vi "CLD3 FGV Timer Exercise.vi"(8 "Fehler (Eingang)":T1, 10 "Zielzeit (s)":dbl, 11 "Timer-Modus":T2) -> (0 "Fehler (Ausgang)":T1, 3 "Verstrichene Zeit (s,ms)":dbl)   [LabVIEW 2009]
doc: "CLD-Übung 3"
uses:
  CLD3 FGV Mode.ctl
panel:
  out "Zeit ist verstrichen":bool
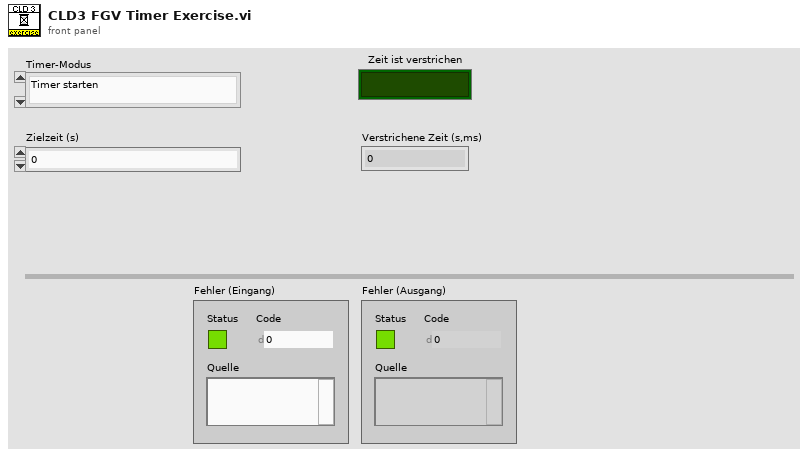
[diagram p1: front panel]
types:
  T1 = cluster{"Status":bool, "Code":i32, "Quelle":string}
  T2 = typedef "CLD3 FGV Mode.ctl" = enum16{"Timer starten", "Zeit lesen", "Anhalten", "Fortsetzen"}
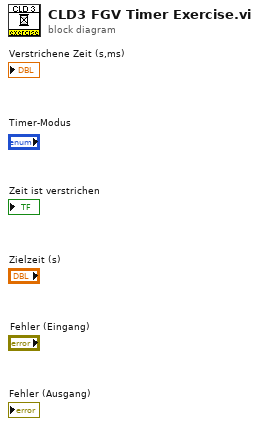
[diagram p0: block diagram]
diagram:
